vi "Write_serial_log.vi"(1 "Log Type":string="SerLog_", 2 "Log Array":string[](array[string]), 3 "Header message":string, 4 "Channel Name":string) -> ()   [LabVIEW 2022 SP3]
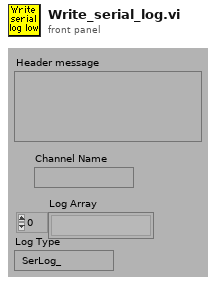
[diagram p1: front panel]
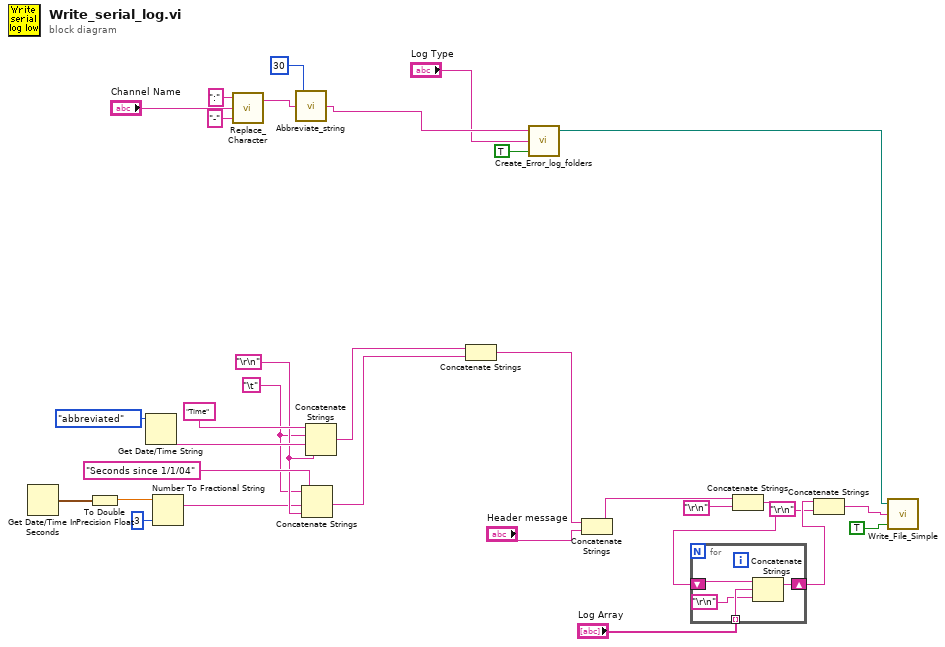
[diagram p0: block diagram]
diagram:
  w8 = "\r\n"
  w3 = "\t"
  n1 = Get Date/Time In Seconds() -> (seconds since 1Jan1904=w4:timestamp)
  n2 = To Double Precision Float(number=w4) -> (double precision float=w7:dbl)
  n3 = Get Date/Time String(date format (0)=enum16{"short", "long", "abbreviated"}."abbreviated") -> (time string=w13:string)  [unwired: 3 out]
  n4 = Number To Fractional String(number=w7, precision (6)=i16 3) -> (F-format string=w5:string)  [unwired: 2 out]
  n5 = call "Replace_Character.vi"("Replace with"="-", "Input String"="Channel Name", "Search For"=":") -> ("Output string"=w20:string)  [unwired: 1 out]
  n6 = call "Abbreviate_string.vi"("Input String"=w20, "Max String Length"=30) -> ("Output String"=w19:string)  [unwired: 1 in, 2 out]
  n7 = Concatenate Strings("Seconds since 1/1/04", w3, w5, w8) -> (w11:string)
  n8 = Concatenate Strings("Time", w3, w13, w8) -> (w12:string)
  n9 = Concatenate Strings(w12, w11) -> (w2:string)
  n10 = call "Create_Error_log_folders.vi"("Log Filename"=w19, "Log Folder"="Log Type", "Per Day Log File?"=TRUE) -> ("Local Log File"=w1:path)  [unwired: 3 in, 1 out]
  n11 = Concatenate Strings(w2, "Header message") -> (w30:string)
  n12 = Concatenate Strings(w30, "\r\n") -> (w28:string)
  n13 = for {
    shift-right: [w34] -> w27
    shift-left: w28 -> [w35]
    tunnel: "Log Array" -> [w33] mode=indexing
    n14 = Concatenate Strings(w35, w33, "\r\n") -> (w34:string)
  }
  n15 = Concatenate Strings(w27, "\r\n") -> (w16:string)
  n16 = call "Write_File_Simple.vi"("append to file? (new file:F)"=TRUE, "character string"=w16, "file path"=w1) -> ()  [unwired: 2 out]
